vi "Send Configuration Load.vi"(7 "Message Priority (Normal)":T1=enum."Normal", 8 "error in":errorcluster, 10 "File Path":path, 11 "Message Enqueuer":refnum<class "Message Enqueuer.lvclass">) -> (0 "error out":errorcluster, 3 "Message Enqueuer out":refnum<class "Message Enqueuer.lvclass">)   [LabVIEW 2018, in "EMS User Interface Actor.lvlib" / "Configuration Load Msg.lvclass"]
uses:
  Configuration Load Msg.lvclass
  <vilib>/ActorFramework/Message Enqueuer/Message Enqueuer.lvclass
  <vilib>/ActorFramework/Message Enqueuer/Message Priority.ctl
  C:/Users/Administrator/Desktop/2018LabVIEW EMS/Dialog Actors/File Dialog Actor/File Dialog Messages/Return File Path Msg/Return File Path Msg.lvclass
  Dialog Actors/File Dialog Actor/File Dialog Messages/Return File Path Msg/Return File Path Msg.lvclass/Return File Path Msg.ctl
  <vilib>/ActorFramework/Message Enqueuer/Message Enqueuer.lvclass/Message Enqueuer.ctl
  <vilib>/ActorFramework/Message Enqueuer/Enqueue.vi
  Dialog Actors/File Dialog Actor/File Dialog Messages/Return File Path Msg/Return File Path Msg.lvclass
  C:/Program Files (x86)/National Instruments/LabVIEW 2018/vi.lib/ActorFramework/Message/Message.lvclass
  <vilib>/ActorFramework/Message Priority Queue/Priority Enqueue.vi
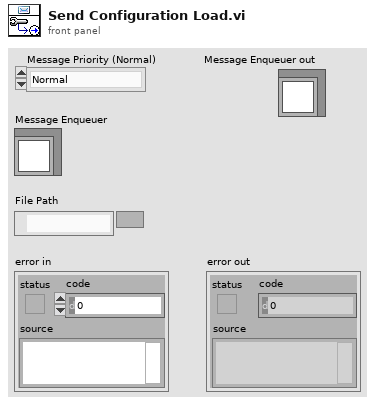
[diagram p1: front panel]
types:
  T1 = typedef "Actor Framework.lvlib/Message Enqueuer.lvclass/Message Priority.ctl" = enum16{"Low", "Normal", "High"}
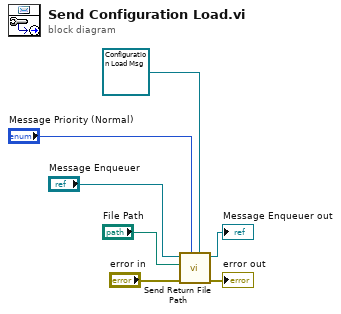
[diagram p0: block diagram]
diagram:
  n1 = call "Send Return File Path.vi"("Message Type"=refnum<class "Configuration Load Msg.lvclass"> refnum ("Master Controller Core.lvlib:Configuration Load Msg.lvclass"), "Message Priority (Normal)"="Message Priority (Normal)", "error in"="error in", "File Path"="File Path", "Message Enqueuer"="Message Enqueuer") -> ("error out"=→"error out":errorcluster, "Message Enqueuer out"=→"Message Enqueuer out":refnum<class "Message Enqueuer.lvclass">)  [unwired: 5 in]
